vi "均匀性最大误差计算.vi"(1 "均匀性表格":string[][](table)=[["A", "O", "E", "O"], ["", "", "", ""], ["", "", "", ""], ["", "", "", ""], ["", "", "", ""], ["", "", "", ""], ["", "", "", ""], ["B", "O", "F", "O"], ["", "", "", ""], ["", "", "", ""], ["", "", "", ""], ["", "", "", ""], ["", "", "", ""], ["", "", "", ""], ["C", "O", "G", "O"], ["", "", "", ""], ["", "", "", ""], ["", "", "", ""], ["", "", "", ""], ["", "", "", ""], ["", "", "", ""], ["D", "O", "H", "O"], ["", "", "", ""], ["", "", "", ""], ["", "", "", ""], ["", "", "", ""], ["", "", "", ""], ["", "", "", ""], ["", "", "", ""], ["", "", "", ""]]) -> (0 "输出数组":string[][](array[string]))   [LabVIEW 2015]
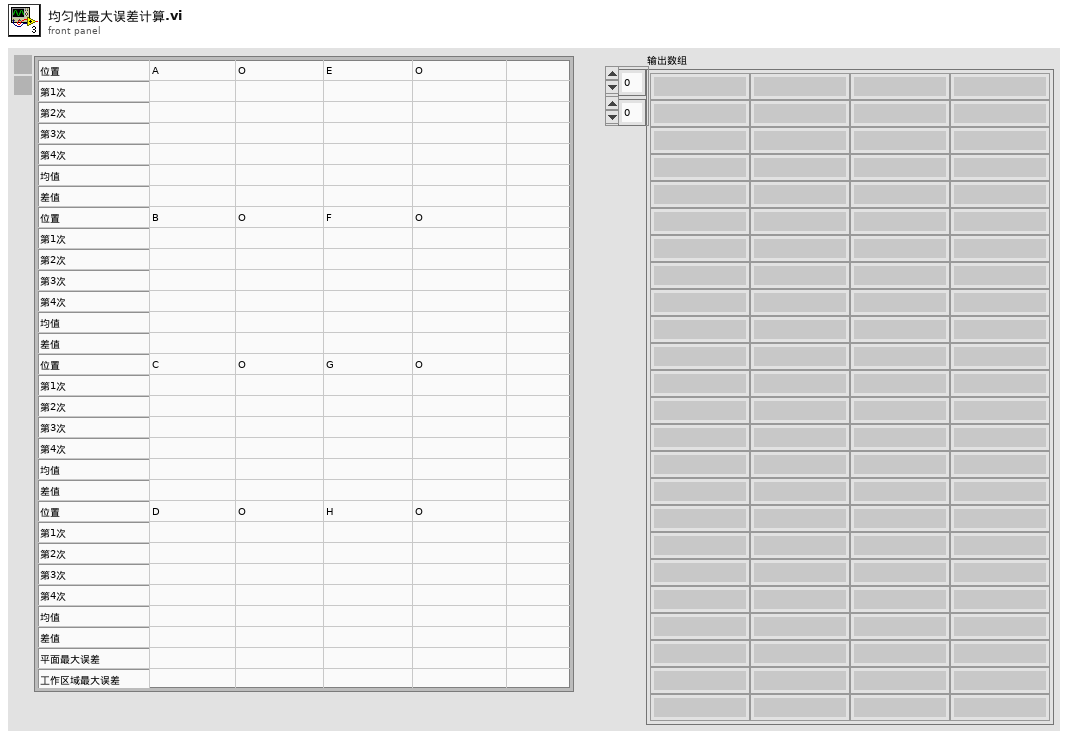
[diagram p1: front panel]
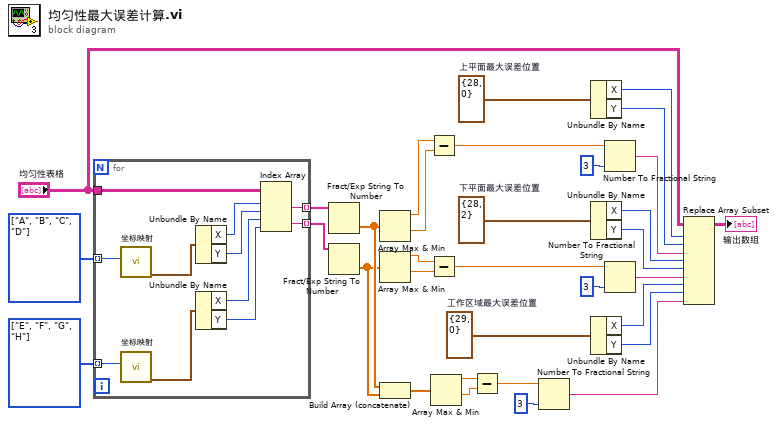
[diagram p0: block diagram]
diagram:
  w5 = cluster{"X":i16, "Y":i16} {"X"=29, "Y"=0}  # 工作区域最大误差位置
  w9 = cluster{"X":i16, "Y":i16} {"X"=28, "Y"=2}  # 下平面最大误差位置
  w13 = cluster{"X":i16, "Y":i16} {"X"=28, "Y"=0}  # 上平面最大误差位置
  w29 = enum16{"A", "B", "C", "D", "E", "F", "G", "H"}[] [enum."E", enum."F", enum."G", enum."H"] items=["A", "B", "C", "D", "E", "F", "G", "H"]
  w33 = enum16{"A", "B", "C", "D", "E", "F", "G", "H"}[] [enum."A", enum."B", enum."C", enum."D"] items=["A", "B", "C", "D", "E", "F", "G", "H"]
  n1 = for {
    tunnel: w33 -> [w44] mode=indexing
    tunnel: "均匀性表格" -> [w42]
    tunnel: [w39] -> w32 mode=indexing
    tunnel: w29 -> [w38] mode=indexing
    tunnel: [w34] -> w28 mode=indexing
    n2 = call "坐标映射.vi"("位置"=w44) -> ("差值坐标"=w43:cluster{"X":i32, "Y":i32})  [unwired: 7 in, 3 out]
    n3 = call "坐标映射.vi"("位置"=w38) -> ("差值坐标"=w37:cluster{"X":i32, "Y":i32})  [unwired: 7 in, 3 out]
    n4 = Unbundle By Name(w43) -> ("X"=w41:i32, "Y"=w40:i32)
    n5 = Unbundle By Name(w37) -> ("X"=w36:i32, "Y"=w35:i32)
    n6 = Index Array(array=w42, index (row) #1=w41, index (col) #1=w40, index (row) #2=w36, index (col) #2=w35) -> (element #1=w39:string, element #2=w34:string)
  }
  n7 = Fract/Exp String To Number(string=w32) -> (number=w21:dbl[])  [unwired: 3 in, 1 out]
  n8 = Fract/Exp String To Number(string=w28) -> (number=w20:dbl[])  [unwired: 3 in, 1 out]
  n9 = Array Max & Min(array=w21) -> (max value=w31:dbl, min value=w30:dbl)  [unwired: 2 out]
  n10 = Array Max & Min(array=w20) -> (max value=w26:dbl, min value=w27:dbl)  [unwired: 2 out]
  n11 = Build Array (concatenate)(w21, w20) -> (w19:dbl[])
  n12 = Subtract(x=w31, y=w30) -> (x-y=w25:dbl)
  n13 = Subtract(x=w26, y=w27) -> (x-y=w24:dbl)
  n14 = Array Max & Min(array=w19) -> (max value=w18:dbl, min value=w17:dbl)  [unwired: 2 out]
  n15 = Subtract(x=w18, y=w17) -> (x-y=w16:dbl)
  n16 = Number To Fractional String(number=w16, precision (6)=i16 3 ("精度(6)")) -> (F-format string=w2:string)  [unwired: 2 in]
  n17 = Unbundle By Name(w13) -> ("X"=w12:i16, "Y"=w11:i16)
  n18 = Unbundle By Name(w9) -> ("X"=w8:i16, "Y"=w7:i16)
  n19 = Unbundle By Name(w5) -> ("X"=w4:i16, "Y"=w3:i16)
  n20 = Number To Fractional String(number=w25, precision (6)=i16 3 ("精度(6)")) -> (F-format string=w10:string)  [unwired: 2 in]
  n21 = Number To Fractional String(number=w24, precision (6)=i16 3 ("精度(6)")) -> (F-format string=w6:string)  [unwired: 2 in]
  n22 = Replace Array Subset(array="均匀性表格", new element #1=w10, index (row) #1=w12, index (col) #1=w11, new element #2=w6, index (row) #2=w8, index (col) #2=w7, new element #3=w2, index (row) #3=w4, index (col) #3=w3) -> (→"输出数组":string[][])
